vi "AskVersion.vi"(8 "error in":errorcluster, 11 "Python":T1) -> (0 "error out":errorcluster, 2 "Version":string, 3 "Python":T1)   [LabVIEW 2022 SP3]
uses:
  PythonCtrl.ctl
  Processors.ctl
panel:
  out "Binary":string
  out "read buffer":string
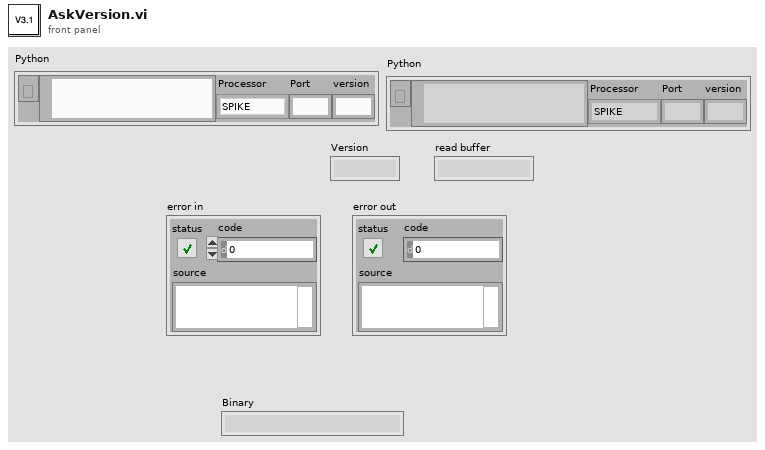
[diagram p1: front panel]
types:
  T1 = typedef "PythonCtrl.ctl" = cluster{"session":refnum<k35>, "PyPath":path, "Processor":T2, "Port":string, "version":string}
  T2 = typedef "Processors.ctl" = enum16{"SPIKE", "Pi", "Pi_ssh", "OpenMV", "Dunio"}
  T3 = enum16{"big-endian, network order", "native, host order", "little-endian"}
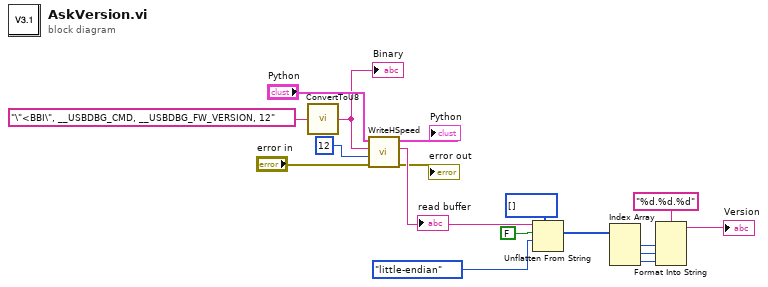
[diagram p0: block diagram]
diagram:
  n1 = call "ConvertToU8.vi"("struct"="\"<BBI\", __USBDBG_CMD, __USBDBG_FW_VERSION, 12" ("write buffer")) -> ("Binary"=w1:string)
  "Binary" <- w1
  n2 = call "WriteHSpeed.vi"("error in"="error in", "Reply length"=12 ("Reply"), "write buffer"=w1, "Python"="Python") -> ("error out"=→"error out":errorcluster, "read buffer"=w13:string, "Python"=→"Python":T1)  [unwired: 5 in]
  "read buffer" <- w13
  n3 = Unflatten From String(type=i32[] [], binary string=w13, data includes array or string size? (T)=FALSE ("prepend array or string size? (T)"), byte order (0:big-endian, network order)=T3."little-endian") -> (value=w10:i32[])  [unwired: 1 in, 2 out]
  n4 = Index Array(array=w10) -> (element #1=w9:i32, element #2=w7:i32, element #3=w6:i32)  [unwired: 3 in]
  n5 = Format Into String(format string="%d.%d.%d", w9, w7, w6) -> (resulting string=→"Version":string)  [unwired: 2 in, 1 out]
